vi "resample to 256by256.vi"(11 "Array":i16[][](array[numeric])) -> (3 "Image Pixels (Float)":i16[][](array[numeric]))   [LabVIEW 2012]
uses:
  <vilib>/vision/NI_Vision_Development_Module.lvlib
panel:
  out "Numeric Control":i32
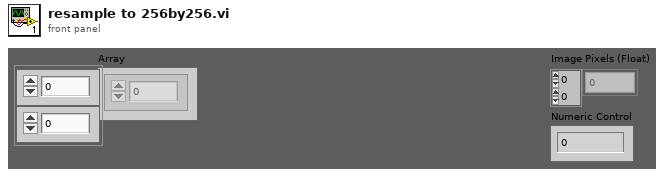
[diagram p1: front panel]
types:
  T1 = typedef "IMAQ Image.ctl" = refnum<image>
  T2 = typedef "Image Type" = u32
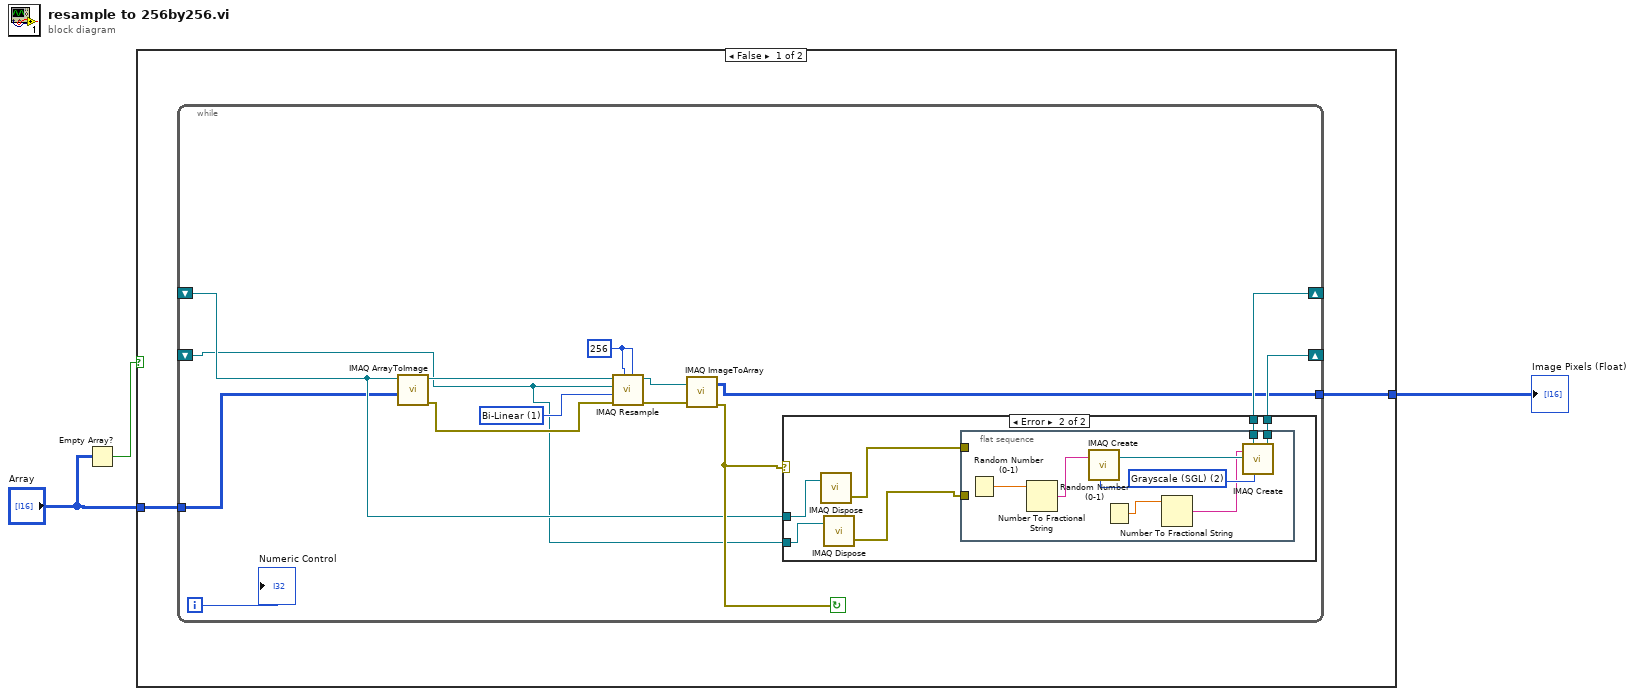
[diagram p0: block diagram]
diagram:
  n1 = Empty Array?(array="Array") -> (empty?=w1:bool)
  n2 = case shown="False" w1 {
    tunnel: "Array" -> [w5 w35]
    tunnel: [w4 w35] -> w3
    frame False {
      n3 = while {
        tunnel: w5 -> [w7]
        shift-right: [w10] -> _
        shift-left: _ -> [w9]
        shift-right: [w11] -> _
        shift-left: _ -> [w12]
        tunnel: [w6] -> w4
        i -> [w8]
        stop <- w13 continue-if-true
        w18 = 256 ("X Resolution")
        w19 = u32 1 items=["Zero Order", "Bi-Linear", "Quadratic", "Cubic Spline"] ("Interpolation Type")
        n4 = call "IMAQ ArrayToImage"("Image Pixels (I16)"=w7, "Image"=w12) -> ("error out"=w15:errorcluster, "Image Out"=w16:T1)  [unwired: 8 in]
        n5 = call "IMAQ Resample"("X Resolution"=w18, "Y Resolution"=w18, "error in (no error)"=w15, "Interpolation Type"=w19, "Image Dst"=w9, "Image Src"=w16) -> ("error out"=w14:errorcluster, "Image Dst Out"=w17:T1)  [unwired: 4 in]
        n6 = call "IMAQ ImageToArray"("error in (no error)"=w14, "Image"=w17) -> ("error out"=w13:errorcluster, "Image Pixels (I16)"=w6:i16[][])  [unwired: 2 in, 3 out]
        n7 = case shown="Error" w13 {
          tunnel: [w21 w27] -> w11
          tunnel: [w20 w26] -> w10
          tunnel: w12 -> [w21 w25]
          tunnel: w9 -> [w20 w23]
          frame No Error {
          }
          frame Error {
            n8 = call "IMAQ Dispose"("Image"=w25) -> ("error out"=w24:errorcluster)  [unwired: 5 in]
            n9 = call "IMAQ Dispose"("Image"=w23) -> ("error out"=w22:errorcluster)  [unwired: 5 in]
            n10 = flat-sequence {
              tunnel: [w34] -> w27
              tunnel: [w33] -> w26
              tunnel: w24 -> [_]
              tunnel: w22 -> [_]
              frame #0 {
                w32 = T2 2 items=["Grayscale (U8)", "Grayscale (I16)", "Grayscale (SGL)", "Complex (CSG)", "RGB (U32)", "HSL (U32)", "RGB (U64)", "Grayscale (U16)"] ("Image Type")
                n11 = Random Number (0-1)() -> (number: 0 to 1=w31:dbl)
                n12 = Number To Fractional String(number=w31) -> (F-format string=w30:string)  [unwired: 3 in]
                n13 = call "IMAQ Create"("Image Name"=w30, "Image Type"=w32) -> ("New Image"=w34:T1)  [unwired: 3 in, 1 out]
                n14 = Random Number (0-1)() -> (number: 0 to 1=w29:dbl)
                n15 = Number To Fractional String(number=w29) -> (F-format string=w28:string)  [unwired: 3 in]
                n16 = call "IMAQ Create"("Image Name"=w28, "Image Type"=w32) -> ("New Image"=w33:T1)  [unwired: 3 in, 1 out]
              }
            }
          }
        }
        "Numeric Control" <- w8
      }
    }
    frame True {
    }
  }
  "Image Pixels (Float)" <- w3
